vi "Start movement.vi"(4 "motor instructions":string, 6 "translation (100)":i32, 7 "forward":bool, 8 "error in (no error)":errorcluster, 9 "period":u32, 10 "initial position (0)":i32, 11 "MotorSim in":refnum<class "MotorSim.lvclass">) -> (0 "error out":errorcluster, 3 "MotorSim out":refnum<class "MotorSim.lvclass">)   [LabVIEW 2018, in "MotorSim.lvclass"]
uses:
  MotorSim.lvclass
  MotorSim.lvclass/MotorSim.ctl
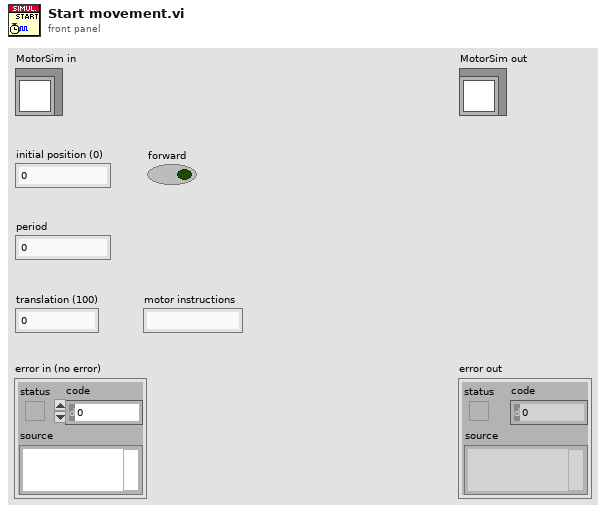
[diagram p1: front panel]
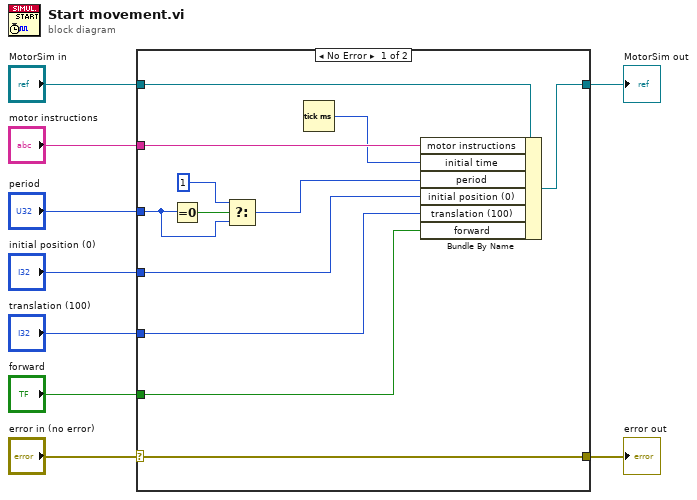
[diagram p0: block diagram]
diagram:
  n1 = case shown="No Error" "error in (no error)" {
    selector: "error in (no error)" -> [w21 w22]
    tunnel: [w21 w22] -> w8
    tunnel: [w19 w23] -> w6
    tunnel: "MotorSim in" -> [w20 w23]
    tunnel: "motor instructions" -> [w17 _]
    tunnel: "forward" -> [w14 _]
    tunnel: "translation (100)" -> [w13 _]
    tunnel: "initial position (0)" -> [w12 _]
    tunnel: "period" -> [w11 _]
    frame No Error {
      n2 = Equal To 0?(x=w11) -> (x = 0?=w16:bool)
      n3 = Select(t=u32 1, s=w16, f=w11) -> (s? t:f=w15:u32)
      n4 = Tick Count (ms)() -> (millisecond timer value=w10:u32)
      n5 = Bundle By Name(cluster=w20, "motor instructions"=w17, "initial time"=w10, "period"=w15, "initial position (0)"=w12, "translation (100)"=w13, "forward"=w14) -> (w19:refnum<class "MotorSim.lvclass">)
    }
    frame Error {
    }
  }
  "error out" <- w8
  "MotorSim out" <- w6
